vi "DAQdemo.vi"() -> ()   [LabVIEW 2016]
panel:
  out "x = y?":bool
  out "波形图":dbl[][](graph)
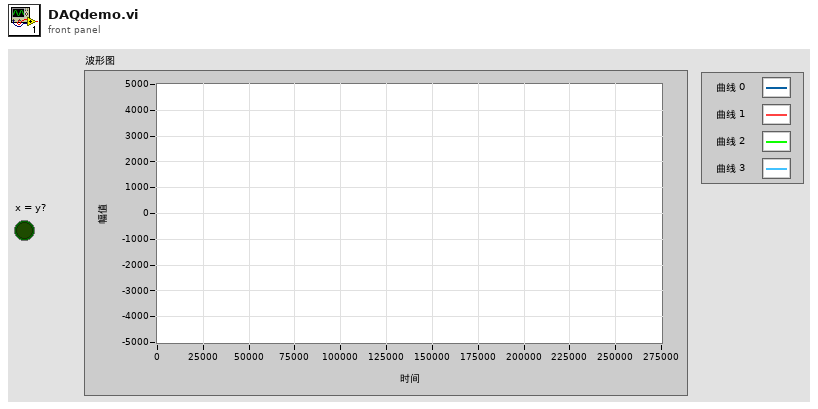
[diagram p1: front panel]
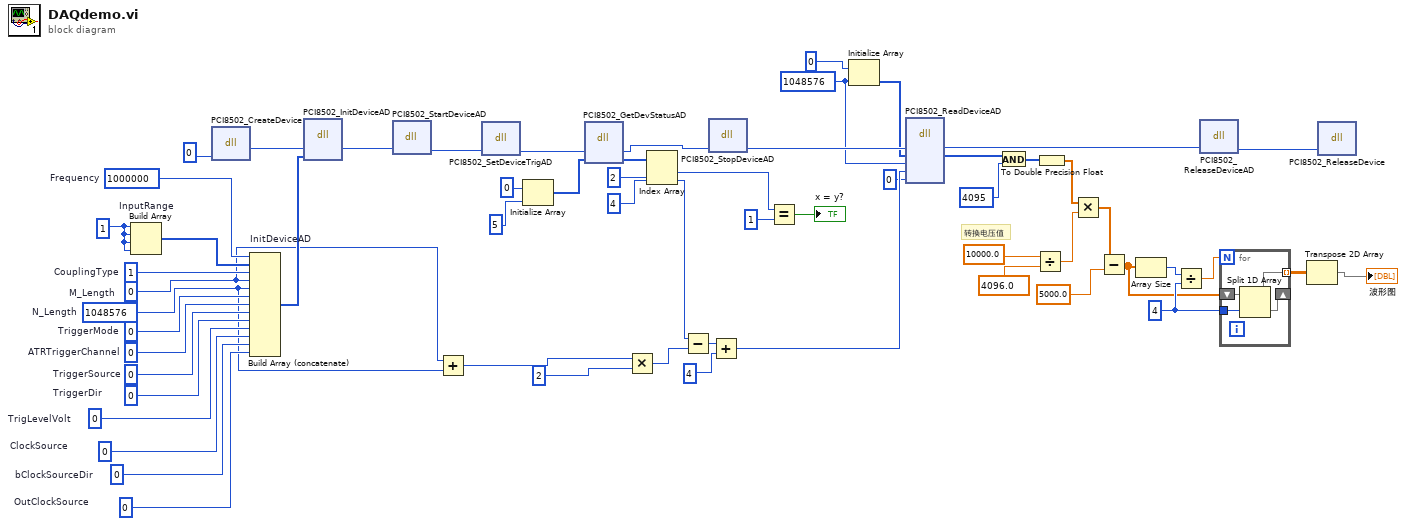
[diagram p0: block diagram]
diagram:
  w9 = 4
  w20 = 1048576 ("dimension size")
  w46 = 0  # OutClockSource
  w47 = 0  # bClockSourceDir
  w48 = 1000000  # Frequency
  w49 = 0  # ClockSource
  w50 = 0  # TrigLevelVolt
  w51 = 1
  w52 = 0  # TriggerDir
  w53 = 0  # TriggerSource
  w54 = 0  # ATRTriggerChannel
  w55 = 0  # TriggerMode
  w25 = 1048576  # N_Length
  w26 = 0  # M_Length
  w56 = 1  # CouplingType
  # "转换电压值"
  n1 = Build Array "InputRange"(w51, w51, w51, w51) -> (w57:i32[])
  n2 = dll-call lib="PTH2aabs F研究\n自制FMCW数据采集阿尔泰采集卡DriverINFamd64PCI8502_32.dll" fn="PCI8502_CreateDevice" label="CreateDevice"("DeviceID"=0) -> ("返回类型"=w58:i32)  [unwired: 4 in, 2 out]
  n3 = Build Array (concatenate) "InitDeviceAD"(w48, w57, w56, w26, w25, w55, w54, w53, w52, w50, w49, w47, w46) -> (w45:i32[])
  n4 = dll-call lib="PTH2aabs F研究\n自制FMCW数据采集阿尔泰采集卡DriverINFamd64PCI8502_32.dll" fn="PCI8502_InitDeviceAD" label="InitDeviceAD"("hDevice"=w58, "pADPara"=w45) -> ("hDevice"=w44:i32)  [unwired: 5 in, 2 out]
  n5 = dll-call lib="PTH2aabs F研究\n自制FMCW数据采集阿尔泰采集卡DriverINFamd64PCI8502_32.dll" fn="PCI8502_StartDeviceAD" label="StartDeviceAD"("hDevice"=w44) -> ("hDevice"=w43:i32)  [unwired: 4 in, 2 out]
  n6 = Add(x=w26, y=w25) -> (x+y=w27:i32)
  n7 = dll-call lib="PCI8502_32" fn="PCI8502_SetDeviceTrigAD" label="SetDeviceTrigAD"("hDevice"=w43) -> ("hDevice"=w40:i32)  [unwired: 4 in, 2 out]
  n8 = Initialize Array(0, 5) -> (w39:i32[])
  n9 = dll-call lib="PTH2aabs F研究\n自制FMCW数据采集阿尔泰采集卡DriverINFamd64PCI8502_32.dll" fn="PCI8502_GetDevStatusAD" label="GetDevStatusAD"("hDevice"=w40, "pADStatus"=w39) -> ("hDevice"=w35:i32, "pADStatus"=w38:i32[])  [unwired: 4 in, 2 out]
  n10 = Multiply(x=w27, y=u32 2) -> (x*y=w29:u32)
  n11 = Index Array(array=w38, index #1=2 ("索引"), index #2=4 ("索引")) -> (element #1=w3:i32, element #2=w24:i32)
  n12 = Subtract(x=w24, y=w29) -> (x-y=w31:u32)
  n13 = dll-call lib="PTH2aabs F研究\n自制FMCW数据采集阿尔泰采集卡DriverINFamd64PCI8502_32.dll" fn="PCI8502_StopDeviceAD" label="StopDeviceAD"("hDevice"=w35) -> ("hDevice"=w34:i32)  [unwired: 4 in, 2 out]
  n14 = Add(x=w31, y=u32 4) -> (x+y=w23:u32)
  n15 = Equal?(x=w3, y=1) -> (x = y?=→"x = y?":bool)
  n16 = Initialize Array(0, w20) -> (w19:i32[])
  n17 = dll-call lib="PTH2aabs F研究\n自制FMCW数据采集阿尔泰采集卡DriverINFamd64PCI8502_32.dll" fn="PCI8502_ReadDeviceAD"("hDevice"=w34, "ADBuffer"=w19, "nReadSizeWords"=w20, "ulStartAddr"=w23, "nRetSizeWords"=0) -> ("hDevice"=w33:i32, "ADBuffer"=w18:u16[])  [unwired: 7 in, 2 out]
  n18 = And(x=w18, y=4095) -> (x .and. y?=w16:i32[])
  n19 = Divide(x=10000.0, y=4096.0) -> (x/y=w12:dbl)
  n20 = To Double Precision Float(number=w16) -> (double precision float=w4:dbl[])
  n21 = Multiply(x=w4, y=w12) -> (x*y=w11:dbl[])
  n22 = Subtract(x=w11, y=5000.0) -> (x-y=w7:dbl[])
  n23 = Array Size(array=w7) -> (size(s)=w10:i32)
  n24 = Divide(x=w10, y=w9) -> (x/y=w8:dbl)
  n25 = dll-call lib="PTH2aabs F研究\n自制FMCW数据采集阿尔泰采集卡DriverINFamd64PCI8502_32.dll" fn="PCI8502_ReleaseDeviceAD" label="ReleaseDeviceAD"("hDevice"=w33) -> ("hDevice"=w32:i32)  [unwired: 4 in, 2 out]
  n26 = for {
    N: w8 -> [_]
    tunnel: w9 -> [w63]
    shift-right: [w61] -> _
    shift-left: w7 -> [w62]
    tunnel: [w60] -> w6 mode=indexing
    n27 = Split 1D Array(array=w62, index=w63) -> (first subarray=w60:dbl[], second subarray=w61:dbl[])
  }
  n28 = Transpose 2D Array(2D array=w6) -> (transposed array=→"波形图":dbl[][])
  n29 = dll-call lib="PTH2aabs F研究\n自制FMCW数据采集阿尔泰采集卡DriverINFamd64PCI8502_32.dll" fn="PCI8502_ReleaseDevice" label="ReleaseDevice"("hDevice"=w32) -> ()  [unwired: 5 in, 2 out]
